vi "Voltage_Divisor.vi"(11 "Voltage":dbl[](array[numeric]) format="%0.2f") -> (3 "Voltage_in":dbl)   [LabVIEW 2013, in "Test_Libraries.lvlib"]
uses:
  Proyecto/Test_Libraries.lvlib
  <vilib>/Analysis/NI_AALBase.lvlib
  <vilib>/Analysis/baseanly.llb/Mean (DBL).vi
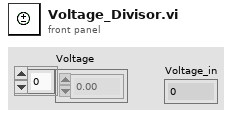
[diagram p1: front panel]
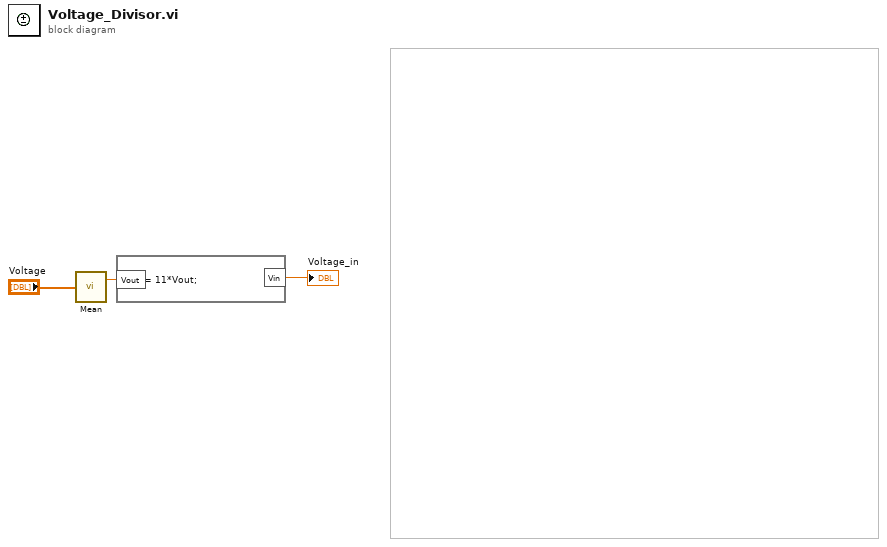
[diagram p0: block diagram]
diagram:
  n1 = call-poly <vilib>:"Mean.vi"("X"="Voltage") -> ("mean"=w3:dbl)  [unwired: 1 out]
  n2 = formula code="Vin = 11*Vout;"("Vout"=w3) -> ("Vin"=→"Voltage_in":dbl)
